vi "Register gRPC Methods.vi"(8 "error in (no error)":errorcluster, 11 "Template Server in":refnum<class "TestDataMarshal.lvclass">) -> (0 "error out":errorcluster, 3 "Template Server out":refnum<class "TestDataMarshal.lvclass">)   [LabVIEW 2019, in "TestDataMarshal.lvlib" / "TestDataMarshal.lvclass"]
uses:
  TestDataMarshal.lvclass
  typeDefs/Server Internal UEs.ctl
  typeDefs/Server Internal Message.ctl
  typeDefs/Server gRPC UEs.ctl
  gRPC lvSupport/Server API/typeDefs/gRPCId Cluster.ctl
  gRPC lvSupport/Server API/typeDefs/grpcId.ctl
  TestDataMarshal.lvclass/TestDataMarshal.ctl
  gRPC lvSupport/gprc-lvsupport.lvlib
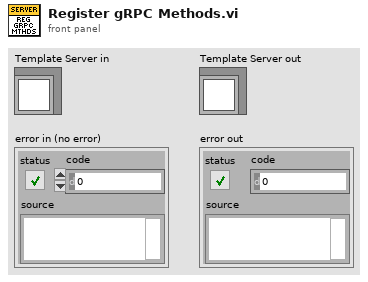
[diagram p1: front panel]
types:
  T1 = typedef "TestDataMarshal.lvlib/TestDataMarshal.lvclass/Server gRPC UEs.ctl" = cluster{"queryserver_QueryServer_Invoke gRPC UE":refnum<user-event>, "queryserver_QueryServer_Query gRPC UE":refnum<user-event>, "queryserver_QueryServer_Register gRPC UE":refnum<user-event>, "queryserver_QueryServer_TestDataTypes gRPC UE":refnum<user-event>}
  T2 = typedef "TestDataMarshal.lvlib/TestDataMarshal.lvclass/Server Internal UEs.ctl" = cluster{"queryserver_QueryServer_Invoke Internal UE":refnum<user-event>, "queryserver_QueryServer_Query Internal UE":refnum<user-event>, "queryserver_QueryServer_Register Internal UE":refnum<user-event>, "queryserver_QueryServer_TestDataTypes Internal UE":refnum<user-event>}
  T3 = typedef "TestDataMarshal.lvlib/gprc-lvsupport.lvlib/grpcId.ctl" = u64
  T4 = typedef "TestDataMarshal.lvlib/TestDataMarshal.lvclass/Server Internal Message UE.ctl" = refnum<user-event>
  T5 = typedef "TestDataMarshal.lvlib/gprc-lvsupport.lvlib/gRPCId Cluster UE.ctl" = refnum<user-event>
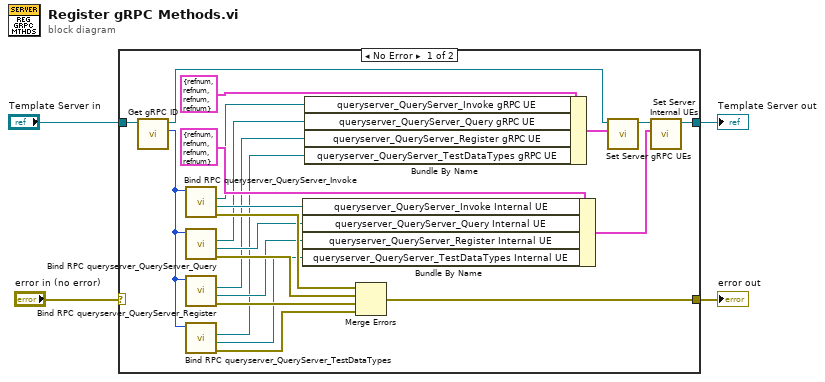
[diagram p0: block diagram]
diagram:
  n1 = case shown="No Error" "error in (no error)" {
    selector: "error in (no error)" -> [_ w27]
    tunnel: "Template Server in" -> [w25 w28]
    tunnel: [w24 w27] -> w3
    tunnel: [w23 w28] -> w2
    frame No Error {
      n2 = call "Get gRPC ID.vi"("OOP Server in"=w25) -> ("gRPC ID"=w17:T3, "OOP Server out"=w26:refnum<class "TestDataMarshal.lvclass">)  [unwired: 9 in]
      n3 = call "Bind RPC queryserver_QueryServer_Invoke.vi"("gRPCid server in"=w17) -> ("error out"=w16:errorcluster, "queryserver_QueryServer_Invoke Internal UE"=w14:T4, "queryserver_QueryServer_Invoke gRPC UE"=w15:T5)  [unwired: 7 in, 1 out]
      n4 = call "Bind RPC queryserver_QueryServer_Query.vi"("gRPCid server in"=w17) -> ("error out"=w13:errorcluster, "queryserver_QueryServer_Query Internal UE"=w11:T4, "queryserver_QueryServer_Query gRPC UE"=w12:T5)  [unwired: 7 in, 1 out]
      n5 = call "Bind RPC queryserver_QueryServer_Register.vi"("gRPCid server in"=w17) -> ("error out"=w10:errorcluster, "queryserver_QueryServer_Register Internal UE"=w8:T4, "queryserver_QueryServer_Register gRPC UE"=w9:T5)  [unwired: 7 in, 1 out]
      n6 = call "Bind RPC queryserver_QueryServer_TestDataTypes.vi"("gRPCid server in"=w17) -> ("error out"=w7:errorcluster, "queryserver_QueryServer_TestDataTypes Internal UE"=w5:T4, "queryserver_QueryServer_TestDataTypes gRPC UE"=w6:T5)  [unwired: 7 in, 1 out]
      n7 = Bundle By Name ("Bundle Internal UEs")(cluster=T2 {"queryserver_QueryServer_Invoke Internal UE"=refnum, "queryserver_QueryServer_Query Internal UE"=refnum, "queryserver_QueryServer_Register Internal UE"=refnum, "queryserver_QueryServer_TestDataTypes Internal UE"=refnum} ("Server Internal UEs"), "queryserver_QueryServer_Invoke Internal UE"=w14, "queryserver_QueryServer_Query Internal UE"=w11, "queryserver_QueryServer_Register Internal UE"=w8, "queryserver_QueryServer_TestDataTypes Internal UE"=w5) -> (w22:T2)
      n8 = Bundle By Name ("Bundle gRPC UEs")(cluster=T1 {"queryserver_QueryServer_Invoke gRPC UE"=refnum, "queryserver_QueryServer_Query gRPC UE"=refnum, "queryserver_QueryServer_Register gRPC UE"=refnum, "queryserver_QueryServer_TestDataTypes gRPC UE"=refnum} ("gRPC Server Method Events"), "queryserver_QueryServer_Invoke gRPC UE"=w15, "queryserver_QueryServer_Query gRPC UE"=w12, "queryserver_QueryServer_Register gRPC UE"=w9, "queryserver_QueryServer_TestDataTypes gRPC UE"=w6) -> (w19:T1)
      n9 = Merge Errors(w16, w13, w10, w7) -> (w24:errorcluster)
      n10 = call "Set Server gRPC UEs.vi"("Server RPC Methods"=w19, "OOP Server in"=w26) -> ("OOP Server out"=w20:refnum<class "TestDataMarshal.lvclass">)  [unwired: 9 in]
      n11 = call "Set Server Internal UEs.vi"("Server Internal UEs"=w22, "OOP Server in"=w20) -> ("OOP Server out"=w23:refnum<class "TestDataMarshal.lvclass">)  [unwired: 9 in]
    }
    frame Error {
    }
  }
  "error out" <- w3
  "Template Server out" <- w2
